vi "PC_ErrorCondition_withrepeatStatesSeek_Test_Sub_VI.vi"(9 "error in":errorcluster, 10 "Path ENI File":path=path "c:/temp/eni.xml" caption="Path ENI File (Create with TwinCAT or EC Engineer)", 11 "IP NIC":string="100.100.100.100") -> (1 "Data values from SC and AC":string, 3 "error out":errorcluster, 8 "Pass":bool)   [LabVIEW 2017]
uses:
  <instrlib>/_Ackermann Automation/EtherCAT Acquisition/ECAT Acq/TypeDefs/ECAT Acq Cluster Activation.ctl
  <instrlib>/_Ackermann Automation/EtherCAT Acquisition/ECAT Acq/ECAT Acq Enum Activation Version.ctl
  <instrlib>/_Ackermann Automation/EtherCAT Acquisition/ECAT Acq/ECAT Acq Enum Bus State Read.ctl
  <instrlib>/_Ackermann Automation/EtherCAT Acquisition/ECAT Acq/ECAT Acq Write PDO Single.vi
  <instrlib>/_Ackermann Automation/EtherCAT Acquisition/ECAT Acq/ECAT Acq Read PDO Single.vi
  <instrlib>/_Ackermann Automation/EtherCAT Acquisition/ECAT Acq/ECAT Acq.lvlib
panel:
  out "Array":string[](array[string])
  out "SC States for Seek with repeat states":dbl[](array[numeric])
  out "Task Ref out":u32
  out "Slave States":T1[](array[typedef])
  out "DC":bool
  out "Activation Data":T2
  in  "Tab":enum32{"Input Data", "Output Data"}(tab)
  out "Variables In":i32[](listbox)
  out "Output Data":u8[](array[numeric]) format="%.0x"
  out "Variables Out":i32(listbox)
  out "Input Data":u8[](array[numeric])
  in  "License Number":string
  out "Count Slaves":u32
  out "Bytes  Output":u32
  in  "Bus Rate Hz":u32=1000
  out "Bytes  Input":u32
  in  "Activation Code":string
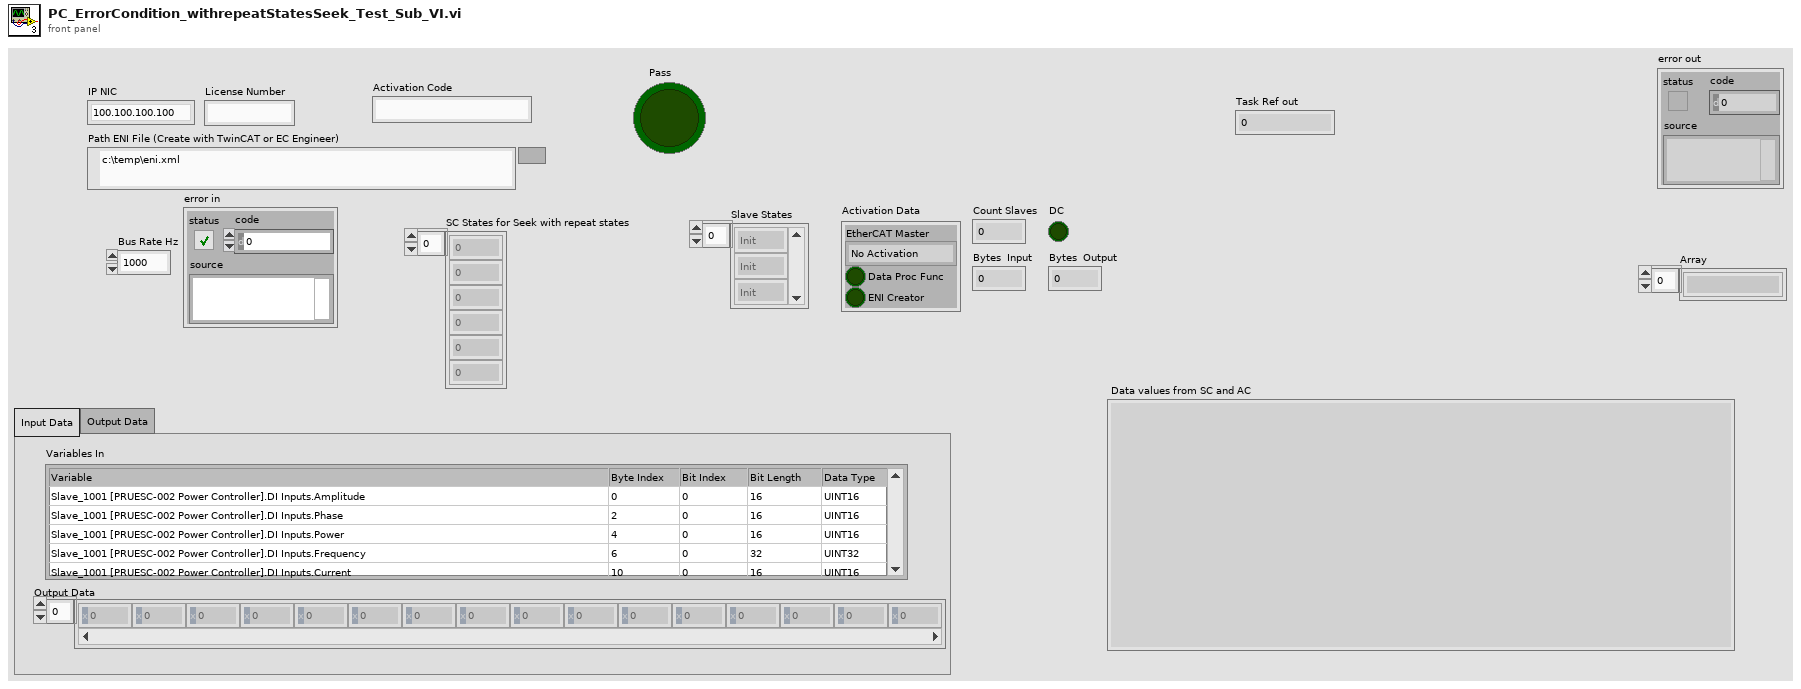
[diagram p1: front panel]
types:
  T1 = typedef "ECAT Acq.lvlib/ECAT Acq Enum Bus State Read.ctl" = enum16{"Init", "PreOp", "Boot", "SafeOp", "Op", "Init Error", "PreOp Error", "Boot Error", "SafeOp Error", "Op Error", "None"}
  T2 = typedef "ECAT Acq.lvlib/ECAT Acq Cluster Activation.ctl" = cluster{"EtherCAT Master":T3, "Data Proc Func":bool, "ENI Creator":bool}
  T3 = typedef "ECAT Acq.lvlib/ECAT Acq Enum Activation Version.ctl" = enum16{"No Activation", "Light", "Standard", "Advanced"}
  T4 = typedef "ECAT Acq.lvlib/ECAT Acq Cluster Bus Setup.ctl" = cluster{"Count Slaves Configured":u32, "PDO Bytes Input":u32, "PDO Bytes Output":u32, "Distributed Clocks":bool}
  T5 = typedef "ECAT Acq.lvlib/ECAT Acq Cluster Process Data Var.ctl" = cluster{"Name":string, "Data Type":T6, "Bit Size":i32, "PDO Index":u16, "Obj Index":u16, "Obj Sub Index":u8, "Byte Index":i32, "Bit Index":i32}
  T6 = typedef "ECAT Acq.lvlib/ECAT Acq Enum Data Types.ctl" = enum16{"Unspecified", "BOOLEAN", "INT8", "INT16", "INT32", "UINT8", "UINT16", "UINT32", "REAL32", "VISIBLE STRING", "OCTET STRING", "UNICODE STRING", "TIME OF DAY", "TIME DIFFERENCE", "Reserved", "DOMAIN", "INT24", "REAL64", "INT40", "INT48", "INT56", "INT64", "UINT24", "No Datatype 1", "UINT40", "UINT48", "UINT56", "UINT64", "No Datatype 3", "No Datatype 4", "PDO Mapping", "No Datatype 5", "Identity", "No Datatype 6", "Command Par", "No Datatype 7", "Sync Par", "No Datatype 8", "0x26", "0x27", "0x28", "0x29", "0x2A", "0x2B", "0x2C", "0x2D", "0x2E", "0x2F", "Bit1", "Bit2", "Bit3", "Bit4", "Bit5", "Bit6", "Bit7", "Bit8"}
  T7 = cluster{"status":bool, "code":i32, "format string":string}
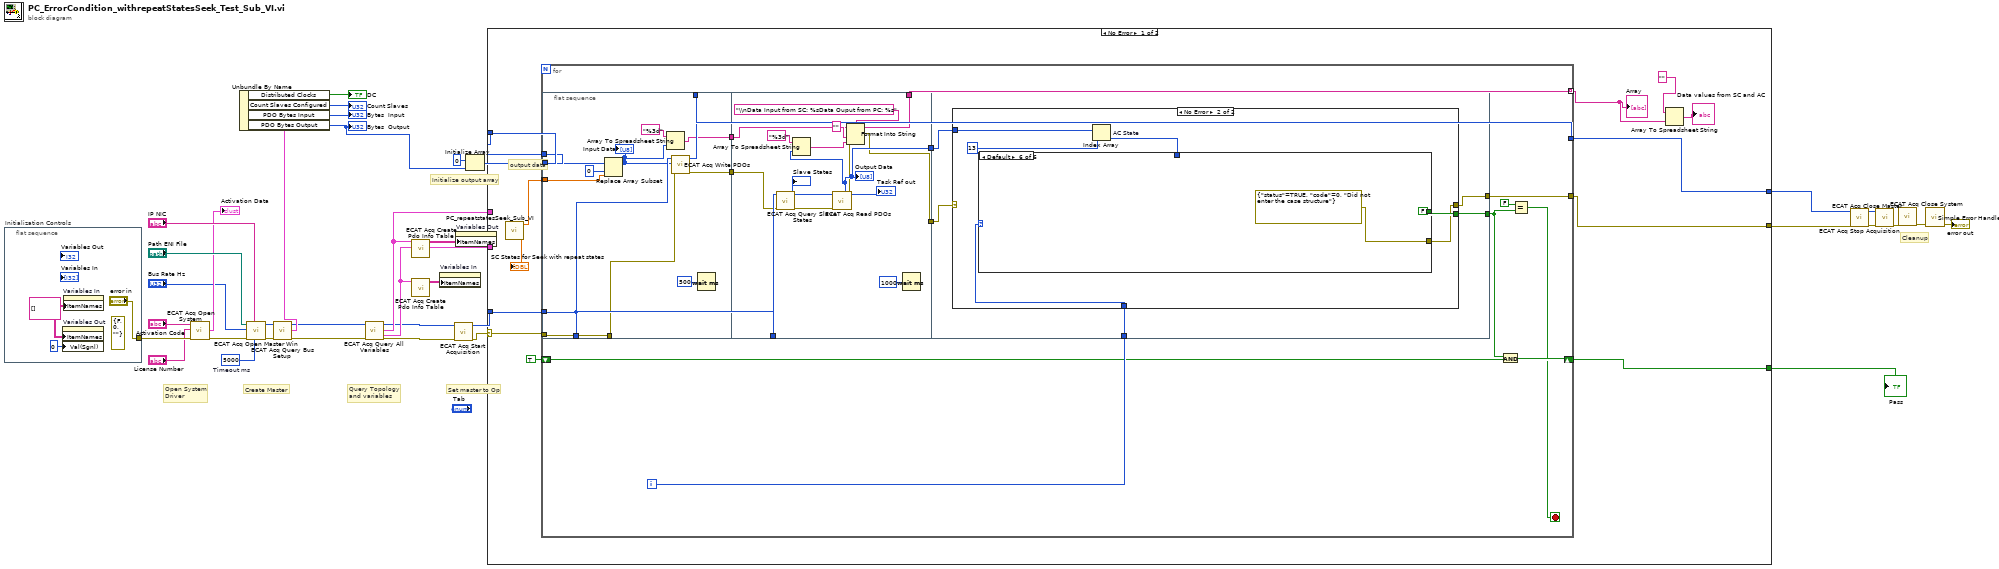
[diagram p0: block diagram]
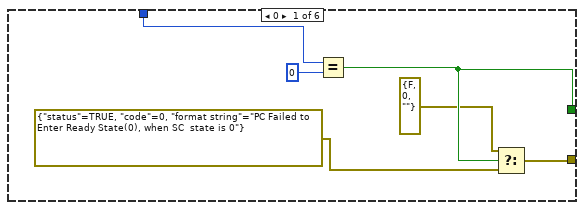
[diagram p3: hidden frame]
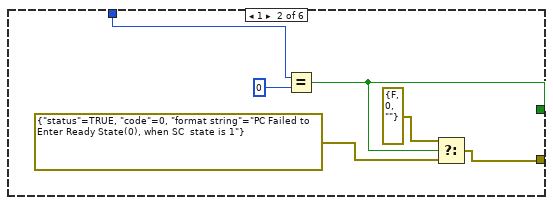
[diagram p4: hidden frame]
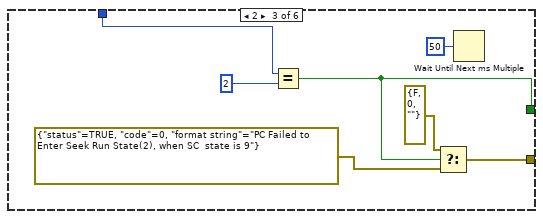
[diagram p5: hidden frame]
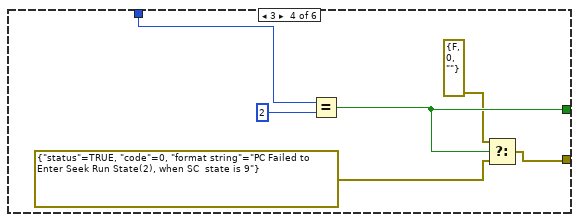
[diagram p6: hidden frame]
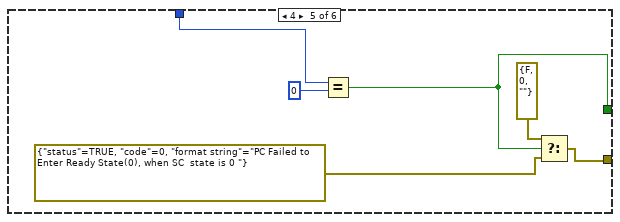
[diagram p7: hidden frame]
diagram:
  w18 = 5000  # Timeout ms
  # "Set master to Op"
  # "Open System\nDriver"
  # "Initialize output array"
  # "Query Topology\nand variables"
  # "Create Master"
  # "Cleanup"
  n1 = flat-sequence "Initialization Controls" {
    tunnel: ["error in"] -> w16
    frame #0 {
      (unwired) errorcluster {"status"=FALSE, "code"=0, "source"=""} ("error in")
      w38 = string[][] [] ("Item Names")
      n2 = property on="Variables Out" class="MCListbox (strict)"("ItemNames"=w38, "Val(Sgnl)"=0 ("Value (Signaling)")) -> ()  [unwired: 2 in, 2 out]
      n3 = property on="Variables In" class="MCListbox (strict)"("ItemNames"=w38) -> ()  [unwired: 2 in, 2 out]
    }
  }
  n4 = call <instrlib>:"ECAT Acq Open System.vi"("error in"=w16, "License Number"="License Number", "Activation Code"="Activation Code") -> ("error out"=w25:errorcluster, "Activation Data"=→"Activation Data":T2)  [unwired: 7 in]
  n5 = call <instrlib>:"ECAT Acq Open Master Win.vi"("Timeout ms"=w18, "IP NIC"="IP NIC", "error in"=w25, "Bus Rate Hz"="Bus Rate Hz", "Path ENI File"="Path ENI File") -> ("error out"=w23:errorcluster, "Task Ref out"=w22:u32)  [unwired: 4 in, 1 out]
  n6 = call <instrlib>:"ECAT Acq Query Bus Setup.vi"("error"=w23, "Task Ref in"=w22) -> ("error out"=w11:errorcluster, "Bus Setup"=w21:T4, "Task ref out"=w14:u32)  [unwired: 7 in]
  n7 = Unbundle By Name(w21) -> ("Distributed Clocks"=→"DC":bool, "Count Slaves Configured"=→"Count Slaves":u32, "PDO Bytes Input"=→"Bytes  Input":u32, "PDO Bytes Output"=w9:u32)
  "Bytes  Output" <- w9
  n8 = call <instrlib>:"ECAT Acq Query All Variables.vi"("error in"=w11, "Task ref"=w14) -> ("error out"=w7:errorcluster, "Variable Entries Inputs"=w35:T5[], "Variable Entries Outputs"=w36:T5[], "Task Ref out"=w10:u32)  [unwired: 6 in]
  n9 = call <instrlib>:"ECAT Acq Create Pdo Info Table.vi"("Variable Entries"=w36) -> ("Table"=w13:string[][])  [unwired: 10 in]
  n10 = call <instrlib>:"ECAT Acq Create Pdo Info Table.vi"("Variable Entries"=w35) -> ("Table"=w12:string[][])  [unwired: 10 in]
  n11 = property on="Variables In" class="MCListbox (strict)"("ItemNames"=w12) -> ()  [unwired: 2 in, 2 out]
  n12 = call <instrlib>:"ECAT Acq Start Acquisition.vi"("error"=w7, "Task Ref in"=w10) -> ("error out"=w1:errorcluster, "Task ref out"=w34:u32)  [unwired: 8 in]
  n13 = property on="Variables Out" class="MCListbox (strict)"("ItemNames"=w13) -> ()  [unwired: 2 in, 2 out]
  n14 = Initialize Array(0 ("element"), w9) -> (w29:i32[])
  n15 = case shown="No Error" w1 {
    selector: w1 -> [w51 w141]
    tunnel: w36 -> [_ _]
    tunnel: w35 -> [_ _]
    tunnel: w34 -> [w48 w142]
    tunnel: w29 -> [w50 _]
    tunnel: [w47 w142] -> w28
    tunnel: [w46 _] -> w4
    tunnel: [w40 w141] -> w3
    frame No Error {
      # "output data"
      n16 = call "PC_repeatstatesSeek_Sub_VI.vi"() -> ("Array"=→"SC States for Seek with repeat states":dbl[], "SC States for Weld"=w45:dbl[])  [unwired: 10 in]
      n17 = for {
        tunnel: w50 -> [w68]
        tunnel: w51 -> [w63]
        shift-right: [w67] -> w46
        shift-left: TRUE -> [w58]
        tunnel: w48 -> [w64]
        tunnel: [w62] -> w47
        tunnel: w45 -> [w57] mode=indexing
        tunnel: [w53] -> w42 mode=indexing
        tunnel: [w52] -> w40
        i -> [w60]
        stop <- w66 stop-if-true
        n18 = flat-sequence {
          tunnel: w68 -> [w79]
          tunnel: w63 -> [w77]
          tunnel: w64 -> [w76]
          tunnel: [w75] -> w62
          tunnel: w57 -> [w73]
          tunnel: [w72] -> w56
          tunnel: [w69] -> w55
          tunnel: w64 -> [w92]
          tunnel: [w87] -> w61
          tunnel: w56 -> [w89]
          tunnel: w55 -> [w84]
          tunnel: [w81] -> w54
          tunnel: [w80] -> w53
          tunnel: w61 -> [w100]
          tunnel: w60 -> [w98]
          tunnel: [w99] -> w59
          tunnel: w54 -> [w97]
          tunnel: [w96] -> w52
          frame #0 {
            n19 = Replace Array Subset(array=w79, new element=w73, index=0) -> (w71:i32[])
            "Input Data" <- w71
            n20 = Array To Spreadsheet String(array=w71, 3:"%3d" ("format string")) -> (spreadsheet string=w69:string)  [unwired: 1 in]
            n21 = call-poly <instrlib>:"ECAT Acq Write PDOs.vi"("error in"=w77, "Output Data"=w71, "Task Ref in"=w76) -> ("error out"=w72:errorcluster, "Task Ref out"=w75:u32)  [unwired: 7 in]
            n22 = Wait (ms)(milliseconds to wait=u32 500) -> ()  [unwired: 1 out]
          }
          frame #1 {
            n23 = call <instrlib>:"ECAT Acq Query Slave States.vi"("error"=w89, "Task Ref in"=w92) -> ("error out"=w94:errorcluster, "Slave States"=→"Slave States":T1[], "Task ref out"=w95:u32)  [unwired: 7 in]
            n24 = call-poly <instrlib>:"ECAT Acq Read PDOs.vi"("error in"=w94, "Task Ref in"=w95) -> ("error out"=w82:errorcluster, "Process Data Input"=w87:u8[], "Task Ref out"=→"Task Ref out":u32)  [unwired: 4 in, 3 out]
            "Output Data" <- w87
            n25 = Array To Spreadsheet String(array=w87, 3:"%3d" ("format string")) -> (spreadsheet string=w85:string)  [unwired: 1 in]
            n26 = Format Into String(format string="\\nData Input from SC: %sData Ouput from PC: %s", initial string="", error in=w82, w84, w85) -> (resulting string=w80:string, error out=w81:errorcluster)
            n27 = Wait (ms)(milliseconds to wait=u32 1000) -> ()  [unwired: 1 out]
          }
          frame #2 {
            n28 = case shown="No Error" w97 {
              selector: w97 -> [w101 _]
              tunnel: w100 -> [_ w106]
              tunnel: [_ w104] -> w99
              tunnel: w98 -> [_ w103]
              tunnel: [w101 w102] -> w96
              frame Error {
              }
              frame No Error {
                n29 = Index Array "AC State"(array=w106, index=13) -> (element=w105:u8)
                n30 = case shown="Default" w103 {
                  tunnel: [w112 w118 w126 w131 w138 FALSE] -> w104
                  tunnel: w105 -> [w111 w117 w123 w130 w136 _]
                  tunnel: [w108 w114 w120 w127 w133 cluster{"status":bool, "code":i32, string} {"status"=TRUE, "code"=0, "Did not enter the case structure"} ("error constant")] -> w102
                  frame 0 {
                    n31 = Equal?(x=w111, y=u8 0) -> (x = y?=w112:bool)
                    n32 = Select(t=errorcluster {"status"=FALSE, "code"=0, "source"=""} ("error constant"), s=w112, f=T7 {"status"=TRUE, "code"=0, "format string"="PC Failed to Enter Ready State(0), when SC  state is 0"} ("error constant")) -> (s? t:f=w108:T7)
                  }
                  frame 1 {
                    n33 = Equal?(x=w117, y=u8 0) -> (x = y?=w118:bool)
                    n34 = Select(t=errorcluster {"status"=FALSE, "code"=0, "source"=""} ("error constant"), s=w118, f=T7 {"status"=TRUE, "code"=0, "format string"="PC Failed to Enter Ready State(0), when SC  state is 1"} ("error constant")) -> (s? t:f=w114:T7)
                  }
                  frame 2 {
                    n35 = Equal?(x=w123, y=u8 2) -> (x = y?=w126:bool)
                    n36 = Select(t=errorcluster {"status"=FALSE, "code"=0, "source"=""} ("error constant"), s=w126, f=T7 {"status"=TRUE, "code"=0, "format string"="PC Failed to Enter Seek Run State(2), when SC  state is 9"} ("error constant")) -> (s? t:f=w120:T7)
                    n37 = Wait Until Next ms Multiple(millisecond multiple=u32 50) -> ()  [unwired: 1 out]
                  }
                  frame 3 {
                    n38 = Equal?(x=w130, y=u8 2) -> (x = y?=w131:bool)
                    n39 = Select(t=errorcluster {"status"=FALSE, "code"=0, "source"=""} ("error constant"), s=w131, f=T7 {"status"=TRUE, "code"=0, "format string"="PC Failed to Enter Seek Run State(2), when SC  state is 9"} ("error constant")) -> (s? t:f=w127:T7)
                  }
                  frame 4 {
                    n40 = Equal?(x=w136, y=u8 0) -> (x = y?=w138:bool)
                    n41 = Select(t=errorcluster {"status"=FALSE, "code"=0, "source"=""} ("error constant"), s=w138, f=T7 {"status"=TRUE, "code"=0, "format string"="PC Failed to Enter Ready State(0), when SC  state is 0 "} ("error constant")) -> (s? t:f=w133:T7)
                  }
                  frame Default {
                  }
                }
              }
            }
          }
        }
        n42 = And(x=w59, y=w58) -> (x .and. y?=w67:bool)
        n43 = Equal?(x=FALSE, y=w59) -> (x = y?=w66:bool)
      }
      "Array" <- w42
      n44 = Array To Spreadsheet String(array=w42, 3:"" ("format string")) -> (spreadsheet string=→"Data values from SC and AC":string)  [unwired: 1 in]
    }
    frame Error {
    }
  }
  "Pass" <- w4
  n45 = call <instrlib>:"ECAT Acq Stop Acquisition.vi"("error"=w3, "Task Ref in"=w28) -> ("error out"=w31:errorcluster, "Task ref out"=w32:u32)  [unwired: 8 in]
  n46 = call <instrlib>:"ECAT Acq Close Master.vi"("error in"=w31, "Task Ref"=w32) -> ("error out"=w30:errorcluster)  [unwired: 9 in]
  n47 = call <instrlib>:"ECAT Acq Close System.vi"("error in"=w30) -> ("error out"=w33:errorcluster)  [unwired: 10 in]
  n48 = call <vilib>:"Simple Error Handler.vi"("error in (no error)"=w33) -> ("error out"=→"error out":errorcluster)  [unwired: 4 in, 4 out]
